vi "Write Current.vi"(8 "error in":errorcluster, 10 "Current":dbl, 11 "IF_XX in":refnum<class "IF_XX.lvclass">) -> (0 "error out":errorcluster, 3 "IF_XX out":refnum<class "IF_XX.lvclass">)   [LabVIEW 2019, in "IF_XX.lvlib" / "IF_XX.lvclass"]
doc: "This routine Sets Current value when the supply is in source mode."
uses:
  Library/IF_XX.lvclass
  C:/Users/Public/Documents/Development/builds/Instruments/PowerSupply.lvlibp/Library/PowerSupply.lvclass
  Library/IF_XX.lvclass/IF_XX.ctl
  builds/Instruments/PowerSupply.lvlibp/Library/PowerSupply.lvclass
panel:
  out "Read data":string
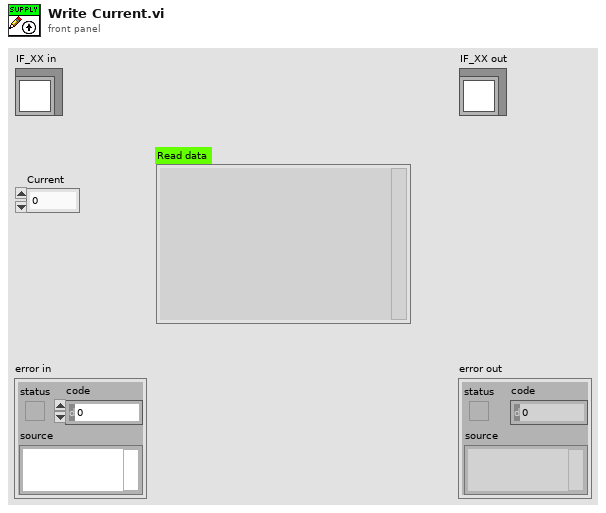
[diagram p1: front panel]
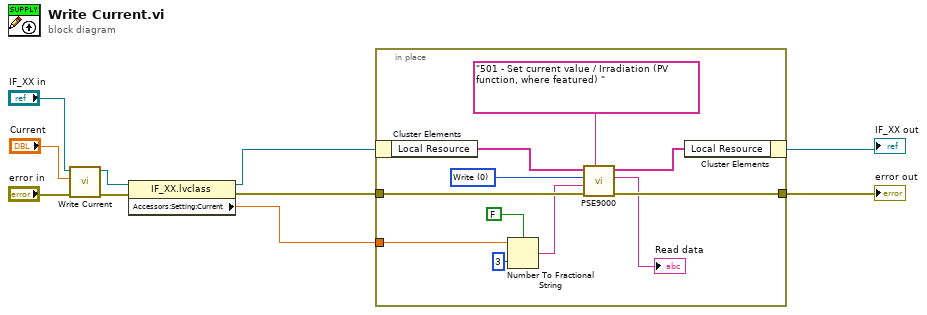
[diagram p0: block diagram]
diagram:
  n1 = call-parent "Write Current.vi"("error in"="error in", "Current"="Current", "PowerSupply in"="IF_XX in") -> ("error out"=w4:errorcluster, "PowerSupply out"=w3:refnum<class "IF_XX.lvclass">)  [unwired: 7 in]
  n2 = property class="IF_XX.lvclass"(reference=w3, error in=w4) -> (reference out=w5:refnum<class "IF_XX.lvclass">, error out=w6:errorcluster, "Accessors:Setting:Current"=w7:dbl)
  n3 = in-place {
    in-place-border: w6 -> [w21]
    in-place-border: [w20] -> w1
    in-place-border: w7 -> [w15]
    w13 = u8 0 items=["Write", "Read"] ("Access")
    n4 = in-place-cluster #1(w5) -> ("Local Resource"=w19:string[])
    n5 = Number To Fractional String(use system decimal point (T)=FALSE, number=w15, precision (6)=i16 3 ("Genauigkeit (6)")) -> (F-format string=w14:string)  [unwired: 1 in]
    n6 = call <instrlib>:"PSE9000.vi"("Command list"="501 - Set current value / Irradiation (PV function, where featured) ", "Error in"=w21, "Value"=w14, "Access"=w13, "Device information in"=w19) -> ("Error out"=w20:errorcluster, "Read data"=→"Read data":string, "Device information out"=w18:string[])  [unwired: 1 in, 1 out]
    n7 = in-place-cluster #1("Local Resource"=w18) -> (→"IF_XX out":refnum<class "IF_XX.lvclass">)
  }
  "error out" <- w1
